vi "Get Participant ID and Input method.vi"(11 "File name":string) -> (2 "Input method":string, 3 "Participant ID":string)   [LabVIEW 2025]
uses:
  <vilib>/regexp/Match Regular Expression.xnode
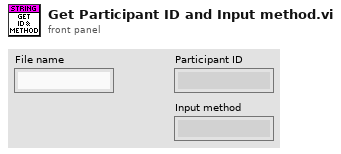
[diagram p1: front panel]
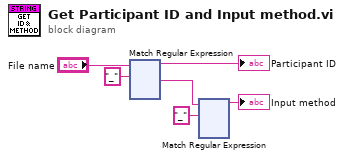
[diagram p0: block diagram]
diagram:
  n1 = xnode "Match Regular Expression"("input string"="File name", "regular expression"="_") -> ("before match"=→"Participant ID":string, "after match"=w3:string)  [unwired: 4 in, 3 out]
  n2 = xnode "Match Regular Expression"("input string"=w3, "regular expression"="_") -> ("before match"=→"Input method":string)  [unwired: 4 in, 4 out]
